vi "Check ACQ Status.vi"(0 "device session in":refnum<class "Device Session.lvclass">, 5 "record number":u64, 11 "error in":errorcluster, 12 "channel":u8=1) -> (3 "record status":T2, 4 "device session out":refnum<class "Device Session.lvclass">, 10 "records done":u64, 13 "overflow occurred":bool, 14 "current record status":T1, 15 "error out":errorcluster)   [LabVIEW 2021, in "Device Session.lvclass"]
doc: "Checks the overall status of the device and reports whether it is operating correctly. This VI checks for system monitor alarms, such as temperature error, power error, FPGA voltage errors, clock PLL lock errors, and channel overload errors.\n\n<B>Input Parameters</B>\n\n<B>device session in</B> is a reference to the Device Session object, which contains a session to each instrument design library used in this sample project. This parameter is obtained from the 'Open Session' VI.\n\n<B>error in</B> describes error conditions that occur before this node runs. This input provides standard 'error in' functionality.\n\n<B>Output Parameters</B>\n\n<B>device session out</B> passes a reference to the session to the next VI.\n\n<B>error out</B> contains error information. This output provides standard 'error out' functionality."
uses:
  Device Session.lvclass
  <instrlib>/_niInstr/Multirecord Acquisition/Interface/v1/Host/Public/Full Record Status.ctl
  <instrlib>/_niInstr/Multirecord Acquisition/Interface/v1/Host/Public/Record State.ctl
  <instrlib>/_niInstr/Multirecord Acquisition/Interface/v1/Host/Public/Record Status.ctl
  Device Session.lvclass/Device Session.ctl
  <instrlib>/_niInstr/Multirecord Acquisition/Interface/v1/Host/niInstr Multirecord Acquisition v1 Host.lvclass
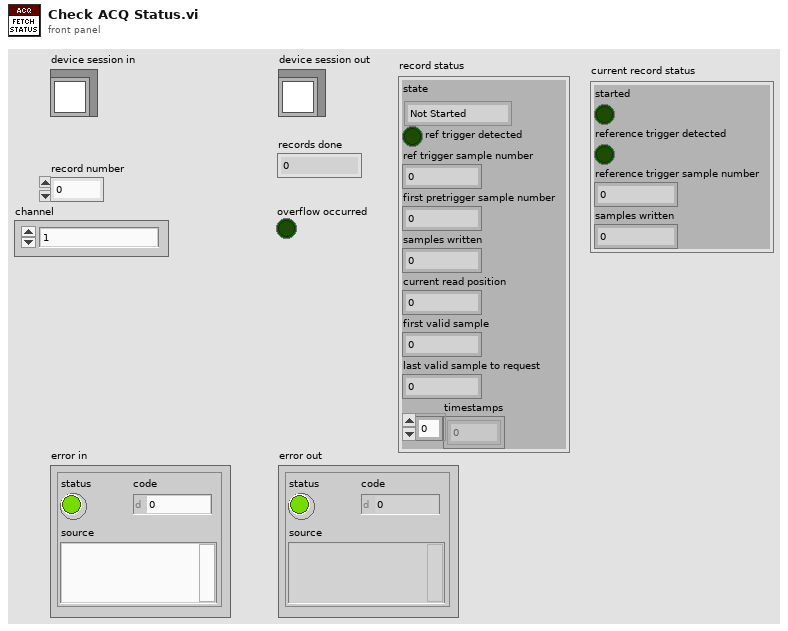
[diagram p1: front panel]
types:
  T1 = typedef "niInstr Multirecord Acquisition v1 Host.lvclass/Record Status.ctl" = cluster{"started":bool, "reference trigger detected":bool, "reference trigger sample number":u64, "samples written":u64}
  T2 = typedef "niInstr Multirecord Acquisition v1 Host.lvclass/Full Record Status.ctl" = cluster{"state":T3, "ref trigger detected":bool, "ref trigger sample number":u64, "first pretrigger sample number":u64, "samples written":u64, "current read position":u64, "first valid sample":u64, "last valid sample to request":u64, "timestamps":u64[]}
  T3 = typedef "niInstr Multirecord Acquisition v1 Host.lvclass/Record State.ctl" = enum16{"Not Started", "Being Acquired", "Completed", "Overwritten"}
  T4 = typedef "Device Session.lvclass/Device Session Object.ctl" = cluster{"fpga reference":T5, "reg bus":refnum<class "niInstr FIFO Register Bus v1 Host.lvclass">, "subsystem map":refnum<class "niInstr Subsystem Map v1 Host.lvclass">, "cal data":refnum<class "niHSAI Cal Data v1 Host.lvclass">, "config":refnum<class "niHSAI Group A Config v1 Host.lvclass">, "acquisition 0":refnum<class "niInstr Multirecord Acquisition v1 Host.lvclass">, "acquisition 1":refnum<class "niInstr Multirecord Acquisition v1 Host.lvclass">, "number of selected acq channels":u8, "selected acq channels":bool[], "number of channels":u32, "configured channels":bool[], "acq configuration":cluster{"number of samples":u64, "number of records":u64, "pretrigger samples":u64}, "actual channel configuration":T6[], "sample clock rate (Hz)":dbl, "scaling coefficients":T10[]}
  T5 = typedef "Device Session.lvclass/FPGA Refnum.ctl" = refnum<k20>
  T6 = typedef "niHSAI Types v1 Host.lvlib/Channel Configuration.ctl" = cluster{"channel":u32, "coupling":T7, "impedance":T8, "bandwidth":T9, "vertical range":dbl, "vertical offset":dbl}
  T7 = typedef "niHSAI Types v1 Host.lvlib/Coupling.ctl" = enum8{"Default", "DC", "AC"}
  T8 = typedef "niHSAI Types v1 Host.lvlib/Impedance.ctl" = enum8{"Default", "1 mega ohm", "50 ohm"}
  T9 = typedef "niHSAI Types v1 Host.lvlib/Bandwidth.ctl" = enum8{"Default", "Full Bandwidth", "Anti-alias Filter", "150 MHz"}
  T10 = typedef "niInstr Multirecord Acquisition v1 Host.lvclass/Scaling Coefficient.ctl" = cluster{"gain":dbl, "offset":dbl}
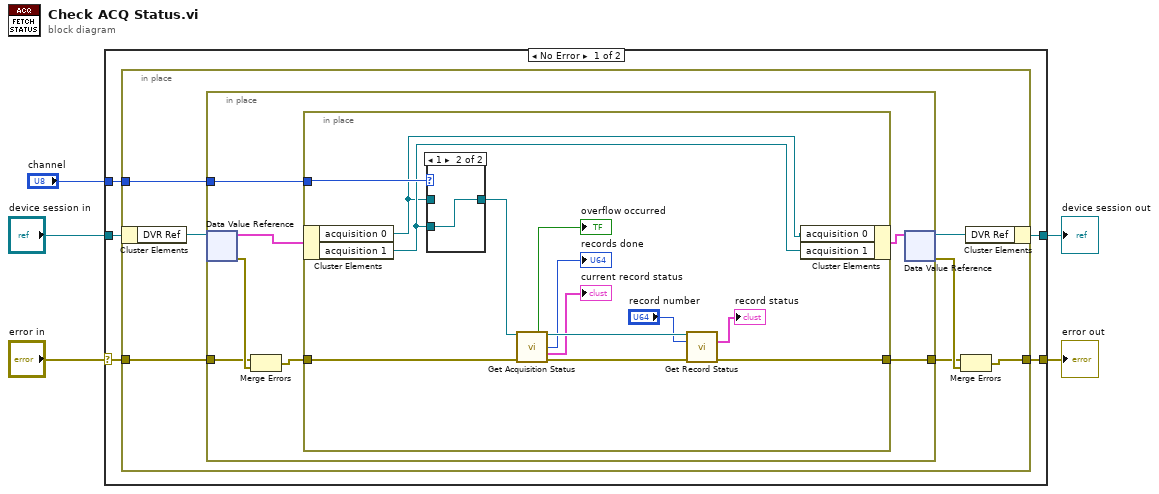
[diagram p0: block diagram]
diagram:
  n1 = case shown="No Error" "error in" {
    selector: "error in" -> [w10 w41]
    tunnel: "device session in" -> [w8 w40]
    tunnel: [w7 w40] -> w3
    tunnel: [w9 w41] -> w2
    tunnel: "channel" -> [w6 _]
    frame No Error {
      n2 = in-place {
        in-place-border: w10 -> [w17]
        in-place-border: [w14] -> w9
        in-place-border: w6 -> [w11]
        n3 = in-place-cluster #1(w8) -> ("DVR Ref"=w13:refnum<data-value>)
        n4 = in-place {
          in-place-border: w17 -> [w21]
          in-place-border: [w24] -> w15
          in-place-border: w11 -> [w18]
          n5 = in-place-dvr #2(w13) -> (w20:T4, w22:errorcluster)
          n6 = Merge Errors(w21, w22) -> (w23:errorcluster)
          n7 = in-place {
            in-place-border: [w36] -> w24
            in-place-border: w23 -> [w37]
            in-place-border: w18 -> [w28]
            n8 = in-place-cluster #3(w20) -> ("acquisition 0"=w26:refnum<class "niInstr Multirecord Acquisition v1 Host.lvclass">, "acquisition 1"=w27:refnum<class "niInstr Multirecord Acquisition v1 Host.lvclass">)
            n9 = case shown="1" w28 {
              tunnel: w27 -> [_ w39]
              tunnel: w26 -> [w38 _]
              tunnel: [w38 w39] -> w25
              frame 0, Default {
              }
              frame 1 {
              }
            }
            n10 = call-dynamic "Get Acquisition Status.vi"("session in"=w25, "error in"=w37) -> ("overflow occurred"=→"overflow occurred":bool, "session out"=w35:refnum<class "niInstr Multirecord Acquisition v1 Host.lvclass">, "records done"=→"records done":u64, "current record status"=→"current record status":T1, "error out"=w34:errorcluster)  [unwired: 8 in, 1 out]
            n11 = call-dynamic "Get Record Status.vi"("session in"=w35, "record number"="record number", "error in"=w34) -> ("record status"=→"record status":T2, "error out"=w36:errorcluster)  [unwired: 10 in, 1 out]
            n12 = in-place-cluster #3("acquisition 0"=w26, "acquisition 1"=w27) -> (w19:T4)
          }
          n13 = in-place-dvr #2(w19) -> (w12:refnum<data-value>, w16:errorcluster)
        }
        n14 = Merge Errors(w15, w16) -> (w14:errorcluster)
        n15 = in-place-cluster #1("DVR Ref"=w12) -> (w7:refnum<class "Device Session.lvclass">)
      }
    }
    frame Error {
    }
  }
  "error out" <- w2
  "device session out" <- w3
